vi "Mono Image-Lookup Table.vi"(8 "error in (no error)":errorcluster, 11 "Image Src":T1) -> (0 "error out":errorcluster, 3 "Image":T1(plugin-control))   [LabVIEW 2016]
uses:
  <vilib>/vision/Image Controls.llb/IMAQ Image.ctl
  <vilib>/vision/NI_Vision_Development_Module.lvlib
panel:
  in  "Operator":T2(ring)=enum."Power X"
  in  "X Value":sgl=25.0 format="%.2f"
  in  "Color":u32(colorbox)=16777222
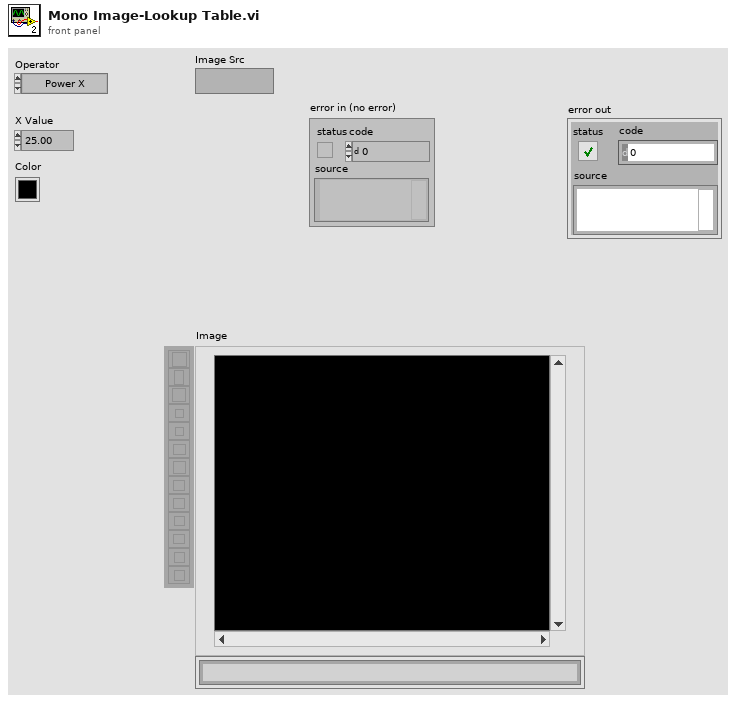
[diagram p1: front panel]
types:
  T1 = typedef "IMAQ Image.ctl" = refnum<image>
  T2 = enum32{"Linear", "Log", "Exp", "Square", "Square root", "Power X", "Power 1/X"}
  T3 = cluster{"Left":i32, "Top":i32, "Right":i32, "Bottom":i32}
  T4 = typedef "Image Type" = u32
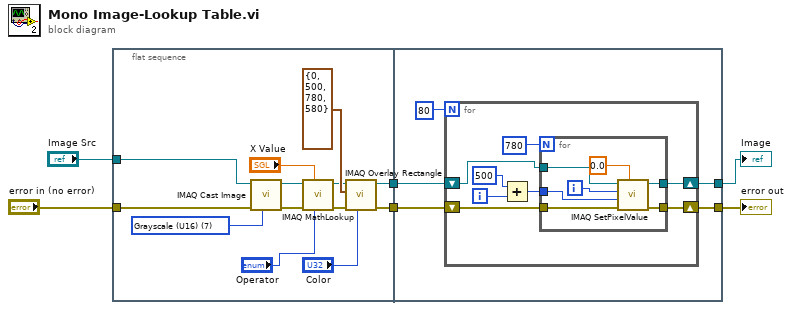
[diagram p0: block diagram]
diagram:
  n1 = flat-sequence {
    tunnel: [w11] -> w6
    tunnel: [w9] -> w5
    tunnel: "error in (no error)" -> [w8]
    tunnel: "Image Src" -> [w7]
    tunnel: w6 -> [w24]
    tunnel: w5 -> [w22]
    tunnel: [w21] -> w2
    tunnel: [w20] -> w4
    frame #0 {
      w19 = T4 7 items=["Grayscale (U8)", "Grayscale (I16)", "Grayscale (SGL)", "Complex (CSG)", "RGB (U32)", "HSL (U32)", "RGB (U64)", "Grayscale (U16)"] ("Image Type")
      n2 = call "IMAQ Cast Image"("Image Type"=w19, "error in (no error)"=w8, "Image Src"=w7) -> ("error out"=w18:errorcluster, "Image Dst Out"=w10:T1)  [unwired: 7 in]
      n3 = call "IMAQ MathLookup"("Operator"="Operator", "X Value"="X Value", "error in (no error)"=w18, "Image Src"=w10) -> ("error out"=w15:errorcluster, "Image Dst Out"=w12:T1)  [unwired: 6 in]
      n4 = call "IMAQ Overlay Rectangle"("Color"="Color", "error in (no error)"=w15, "Rectangle"=T3 {"Left"=0, "Top"=500, "Right"=780, "Bottom"=580}, "Image"=w12) -> ("error out"=w9:errorcluster, "Image Out"=w11:T1)  [unwired: 6 in]
    }
    frame #1 {
      n5 = for {
        N: 80 -> [_]
        shift-right: [w30] -> w20
        shift-left: w22 -> [w31]
        shift-right: [w29] -> w21
        shift-left: w24 -> [w28]
        i -> [w27]
        n6 = Add(x=500, y=w27) -> (x+y=w25:i32)
        n7 = for {
          N: 780 ("Numeric") -> [_]
          tunnel: w31 -> [w38]
          tunnel: [w37] -> w30
          tunnel: w28 -> [w35]
          tunnel: [w34] -> w29
          tunnel: w25 -> [w33]
          i -> [w39]
          n8 = call "IMAQ SetPixelValue"("Pixel Value"=sgl 0.0, "error in (no error)"=w38, "Y Coordinate"=w33, "X Coordinate"=w39, "Image"=w35) -> ("error out"=w37:errorcluster, "Image Out"=w34:T1)  [unwired: 5 in]
        }
      }
    }
  }
  "error out" <- w4
  "Image" <- w2
